vi "PES delay Mihai_March 2 2016 Brett1a.vi"(5 "Set velocity":string="200000") -> ()   [LabVIEW 2016]
uses:
  <vilib>/Waveform/WDTFileIO.llb/Export Waveforms To Spreadsheet File (1D).vi
  <vilib>/Instr/_visa.llb/VISA Configure Serial Port (Instr).vi
  <vilib>/Waveform/WDTFileIO.llb/Export Waveform To Spreadsheet File.vi
panel:
  out "Response 3":string="OK"
  out "Error 4":i32
  in  "Module # 3":i16
  out "Error 2":i32
  in  "Module # 4":i16
  out "Error 3":i32
  out "concatenated string 2":string="MA -21424\r"
  out "number 2":dbl=-21164.0
  out "return count 7":u32=15
  out "concatenated string":string="MA    104762\r"
  out "return count 5":u32=15
  out "read buffer 5":string="P:-0007564095\r\n"
  out "return count 4":u32
  out "return count 3":u32=15
  out "return count":u32
  out "read buffer":string
  in  "Resource Name":refnum<visa-resource-name>="COM1"
  in  "Baud Rate (9600)":u32=9600
  out "Error Information":errorcluster
  out "RoiSum":dbl=1786426.0
  out "ps 2":dbl=9.99159 format="%#_10g"
  out "coerced(x)":dbl=-2.22222
  out "P7887Sts Error":i32
  out "P7887Dat Error":i32
  out "TotalSum":dbl=1790796.0
  out "decimal integer string 2":string="MA -21424"
  out "Steps":dbl=-21423.532738095226 format="%.3f"
  out "mm 2":string="P:-0000021164\r\n"
  in  "offset 2":i32=2
  in  "Module # 2":i16
  out "Response 2":string="OK"
  in  "Tab Control 2":T1(tab)=enum."Measure PES"
  in  "offset":i32=2
  in  "stop":bool
  in  "Tab Control":enum32{"Setings", "Move / Measure"}(tab)=enum."Move / Measure"
  out "String":string="SV200000"
  out "number":dbl=104670.0
  out "go to new":string="    104762"
  out "ps":dbl=10.990350000000001 format="%#_10g"
  in  "ps":dbl=11.0
  out "Steps":dbl=104761.90476190475 format="%.3f"
  out "STEPS":string="P:+0000104670\r\n"
  in  "Radio Buttons":T2(radio)=enum."Radio Selection 4"
  in  "Boolean":bool=TRUE
  out "Status 3":T3={"Running"=1, "Runtime"=200.172, "TotalSum"=1790796.0, "RoiSum"=1786426.0, "RoiRate"=9885.0, "Fifo full"=0.0, "Sweeps"=199118.0, "Start events"=199118.0, "Maxval"=0} {"Fifo full" format="%.2f"; "Sweeps" format="%.2f"; "Start events" format="%.2f"; "RoiRate" format="%.2f"; "RoiSum" format="%.2f"; "TotalSum" format="%.2f"; "Runtime" format="%.2f"}
  in  "Transient Destination":path=path "C:/Documents and Settings/admin/My Documents/PES/2016/160310/T1_800+800nm.txt"
  out "XY Graph":T4(graph)=[{"Current position"=1.77597, "TotalSum"=1804610.0, "RoiSum"=1800421.0}, {"Current position"=1.5232350000000001, "TotalSum"=1788425.0, "RoiSum"=1783863.0}, {"Current position"=1.27617, "TotalSum"=1802098.0, "RoiSum"=1797659.0}, {"Current position"=1.023435, "TotalSum"=1791426.0, "RoiSum"=1786595.0}, {"Current position"=0.7745850000000001, "TotalSum"=1787483.0, "RoiSum"=1782845.0}, {"Current position"=0.52521, "TotalSum"=1821808.0, "RoiSum"=1817193.0}, {"Current position"=0.27604500000000004, "TotalSum"=1814052.0, "RoiSum"=1809669.0}, {"Current position"=0.027615, "TotalSum"=1806153.0, "RoiSum"=1801377.0}, {"Current position"=-0.22995000000000002, "TotalSum"=1812902.0, "RoiSum"=1808127.0}, {"Current position"=-0.47418000000000005, "TotalSum"=1823284.0, "RoiSum"=1818381.0}, {"Current position"=-0.728175, "TotalSum"=1800762.0, "RoiSum"=1796036.0}, {"Current position"=-0.9750300000000001, "TotalSum"=1812486.0, "RoiSum"=1807331.0}, {"Current position"=-1.222305, "TotalSum"=1825573.0, "RoiSum"=1821216.0}, {"Current position"=-1.46937, "TotalSum"=1829525.0, "RoiSum"=1824666.0}, {"Current position"=-1.721055, "TotalSum"=1840480.0, "RoiSum"=1835769.0}, {"Current position"=-1.96938, "TotalSum"=1820091.0, "RoiSum"=1815294.0}]
  out "x-y 2":dbl=-3.991535
  in  "No of steps":sgl=20.0 min=1 step=1
  in  "End":dbl=-10.0
  out "Begin":dbl=1.991535
  out "PS per step":dbl=-0.2494709375 min=1.0 max=10.0 step=1.0 format="%#_8g"
  out "Current position":dbl=-2.22222 format="%#_10g"
  out "appended path":path=path "C:/Documents and Settings/admin/My Documents/PES/2016/160310/2 TO -2 PS/2 TO -2/-2_22E+0.dat"
  in  "Photoelectron Spectra Destination":path=path "C:/Documents and Settings/admin/My Documents/PES/2016/160310/10 to -10/1_02E+0.dat"
  in  "No of Sweeps":dbl=199000.0
  out "Actual":dbl=199118.0
  in  "Module #":i16
  out "Settings P7887":T5={"Range"=6528, "Prena"=16, "Single sweeps"=39321856, "RoiMin"=2000, "RoiMax"=6500, "Roipreset"=0.0, "Timepreset"=1000.0, "SaveData"=0, "Format"=0, "Increm. Name"=FALSE, "Cycles"=2, "Sweep mode"=672, "Sync Out"=768, "Bitshift"=0, "Digval"=0, "Digio"=0, "DAC01"=29568, "DAC23"=31488, "SweepPreset"=200000.0, "#Regions"=0, "Caluse"=1, "First channel"=0.0, "Active"=1, "Calpoints"=0} {"DAC23" format="%.0x"; "DAC01" format="%.0x"; "Digio" format="%.0x"; "Sweep mode" format="%.0x"; "Prena" format="%.0x"; "First channel" format="%.2f"; "Sync Out" format="%.0x"; "SweepPreset" format="%.2f"; "SaveData" format="%.0x"; "Timepreset" format="%.2f"; "Roipreset" format="%.2f"}
  out "Data":u32[](graph)
  out "position set":dbl=-2.249470937499999 min=1.0 max=10.0 step=1.0 format="%#_8g"
  in  "Status":T6(radio)=enum."Finish recorging S#"
  # "Delay"
  # "Delay"
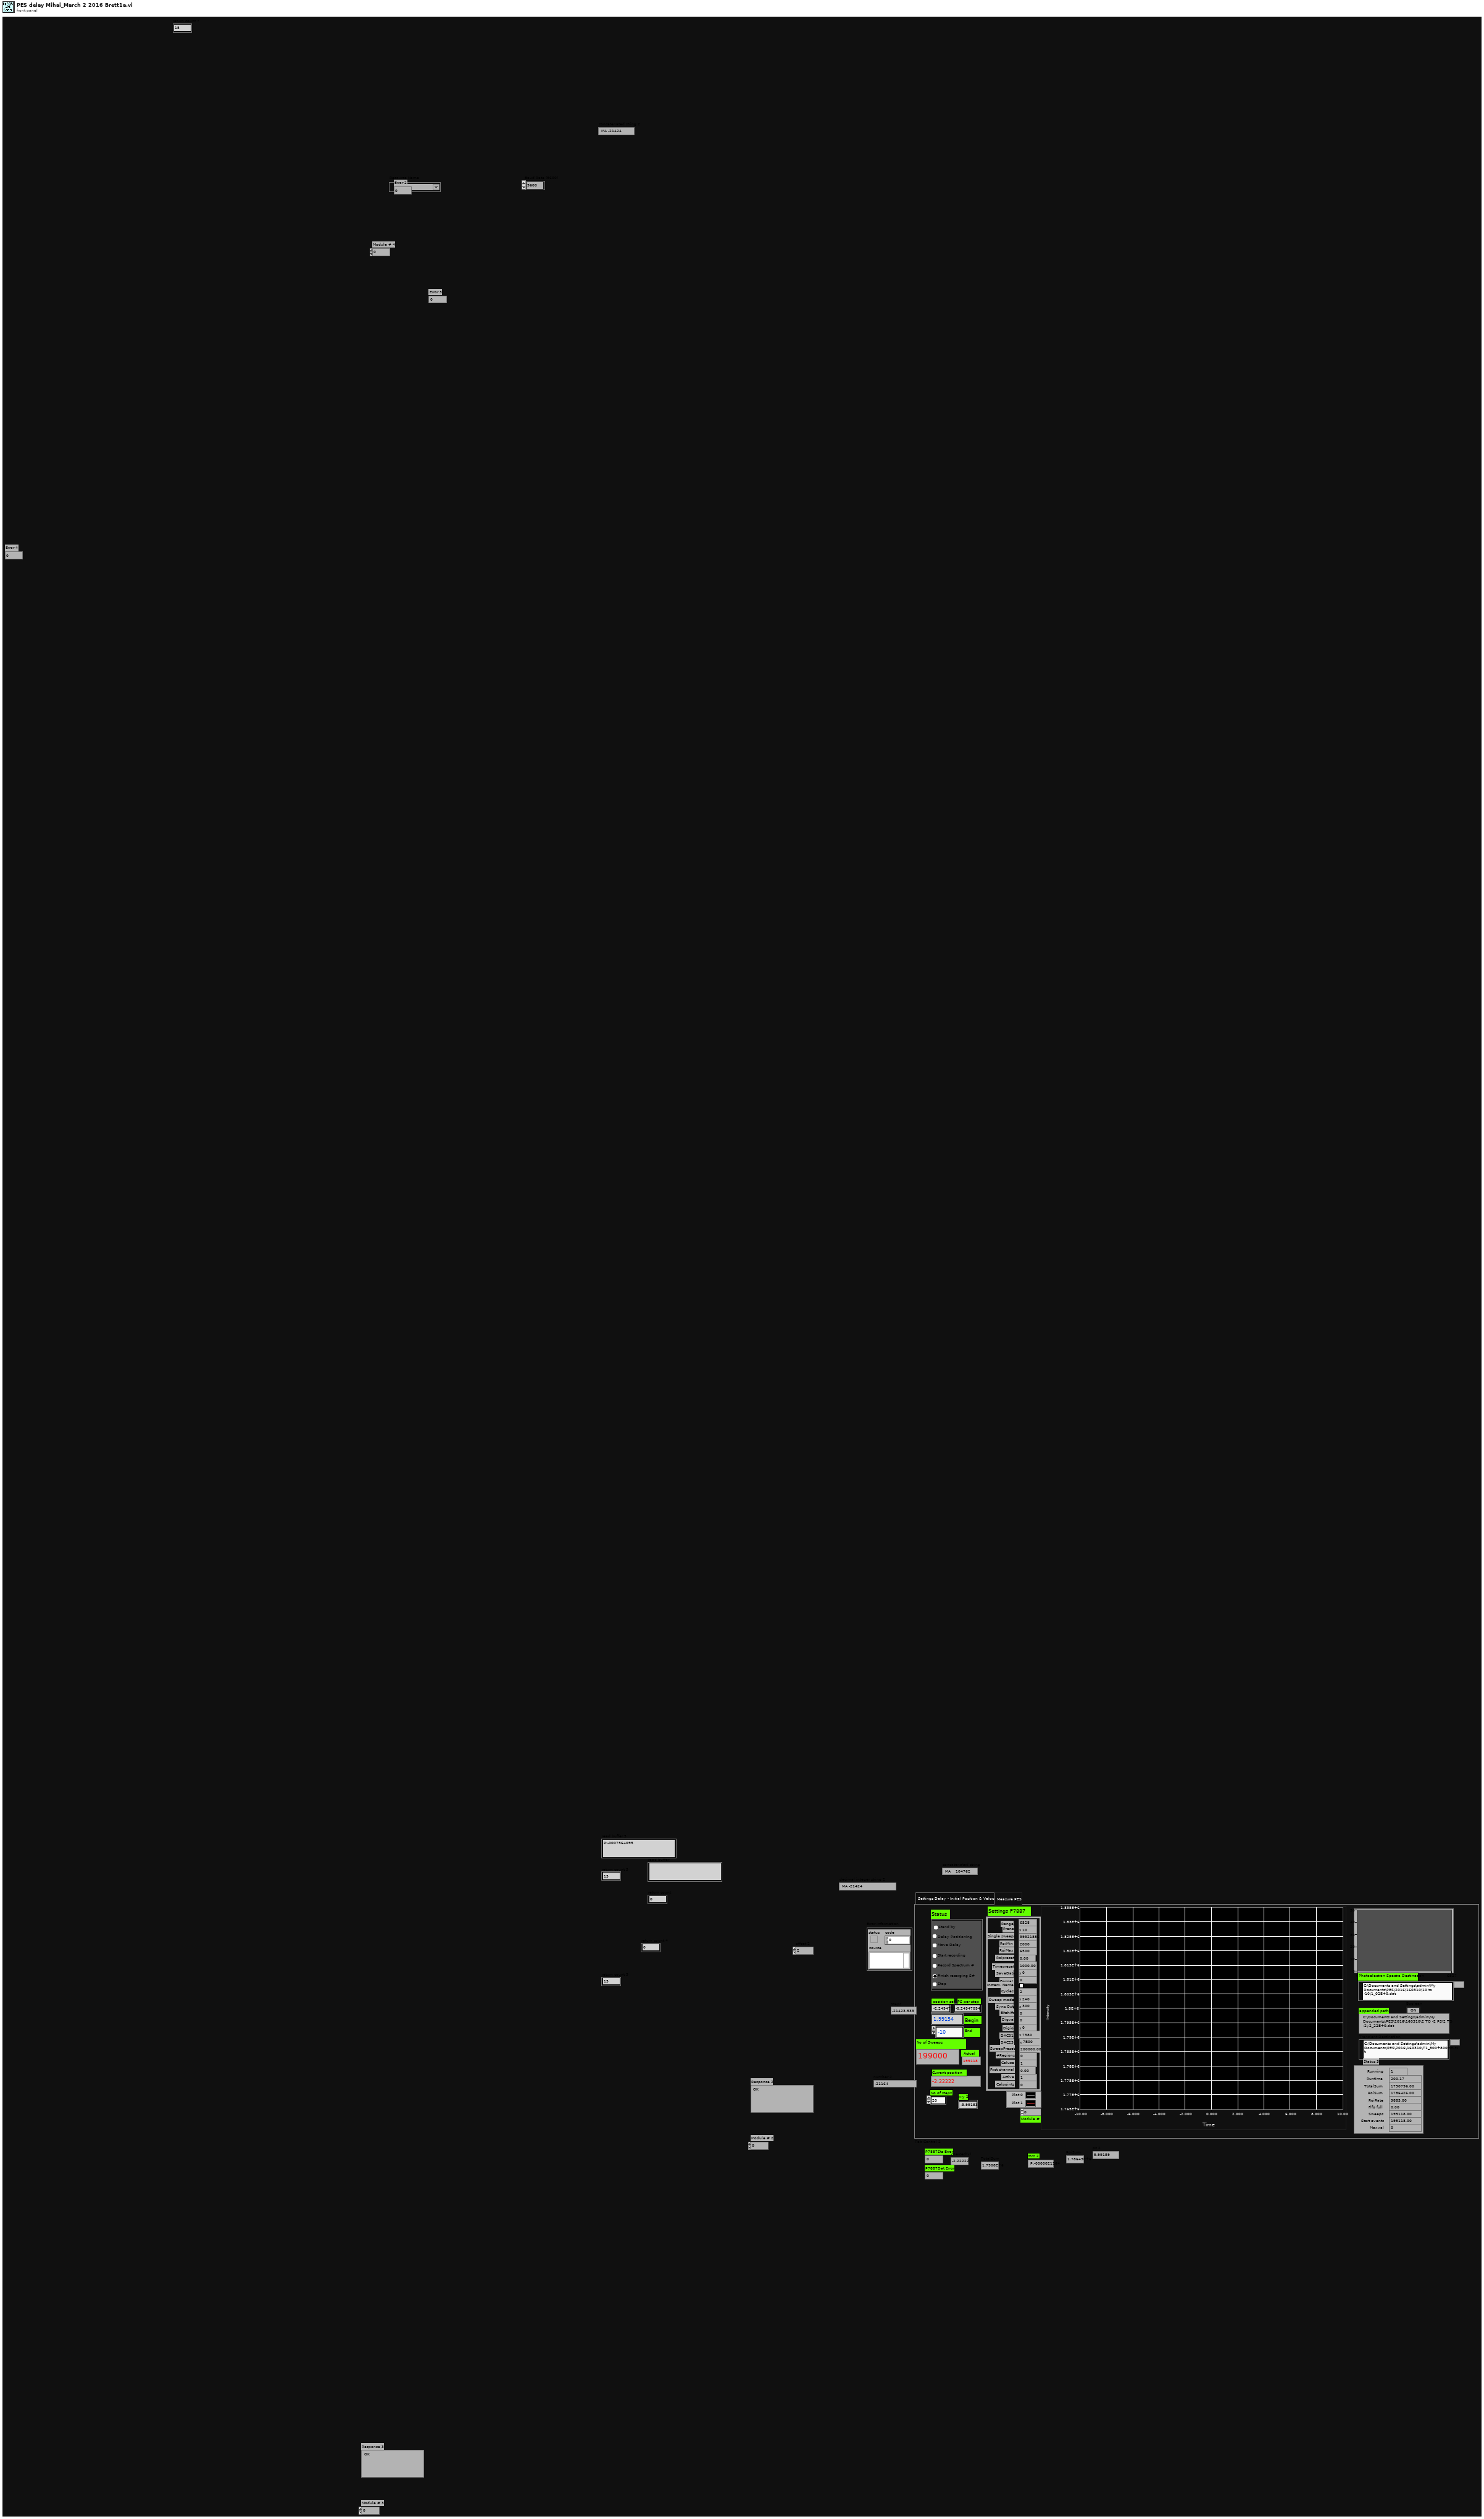
[diagram p1: front panel]
types:
  T1 = enum32{"Settings Delay - Initial Pozition & Velocity", "Measure PES"}
  T2 = enum32{"Stop", "Radio Selection 2", "Radio Selection 3", "Radio Selection 4"}
  T3 = cluster{"Running":i32, "Runtime":dbl, "TotalSum":dbl, "RoiSum":dbl, "RoiRate":dbl, "Fifo full":dbl, "Sweeps":dbl, "Start events":dbl, "Maxval":u32}
  T4 = cluster{"Current position":dbl, "TotalSum":dbl, "RoiSum":dbl}[]
  T5 = cluster{"Range":i32, "Prena":u32, "Single sweeps":u32, "RoiMin":u32, "RoiMax":u32, "Roipreset":dbl, "Timepreset":dbl, "SaveData":u32, "Format":i32, "Increm. Name":bool, "Cycles":u32, "Sweep mode":u32, "Sync Out":u32, "Bitshift":i32, "Digval":u32, "Digio":u32, "DAC01":u32, "DAC23":u32, "SweepPreset":dbl, "#Regions":i32, "Caluse":i32, "First channel":dbl, "Active":i32, "Calpoints":i32}
  T6 = enum32{"Delay Pozitioning", "Move Delay", "Record Spectrum #", "Finish recorging S#", "Stop ", "Start recording", "Stand by"}
  T7 = enum32{"Delay Pozitioning", "Move Delay", "Record Spectrum #", "Finish recorging S#", "Stop", "Start recording", "Stand by"}
  T8 = cluster{"Range":i32, "Prena":u32, "Cftfak":i32, "RoiMin":u32, "RoiMax":u32, "Roipreset":dbl, "Timepreset":dbl, "SaveData":u32, "Format":i32, "Increm. Name":bool, "Cycles":u32, "Sweep mode":u32, "Sync Out":u32, "Bitshift":i32, "Digval":u32, "Digio":u32, "DAC0":u32, "DAC1":u32, "SweepPreset":dbl, "#Regions":i32, "Caluse":i32, "First channel":dbl, "Active":i32, "Calpoints":i32}
  T9 = cluster{"Current position":dbl, "TotalSum":dbl, "RoiSum":dbl}
  T10 = cluster{waveform(dbl), waveform(dbl), waveform(dbl)}
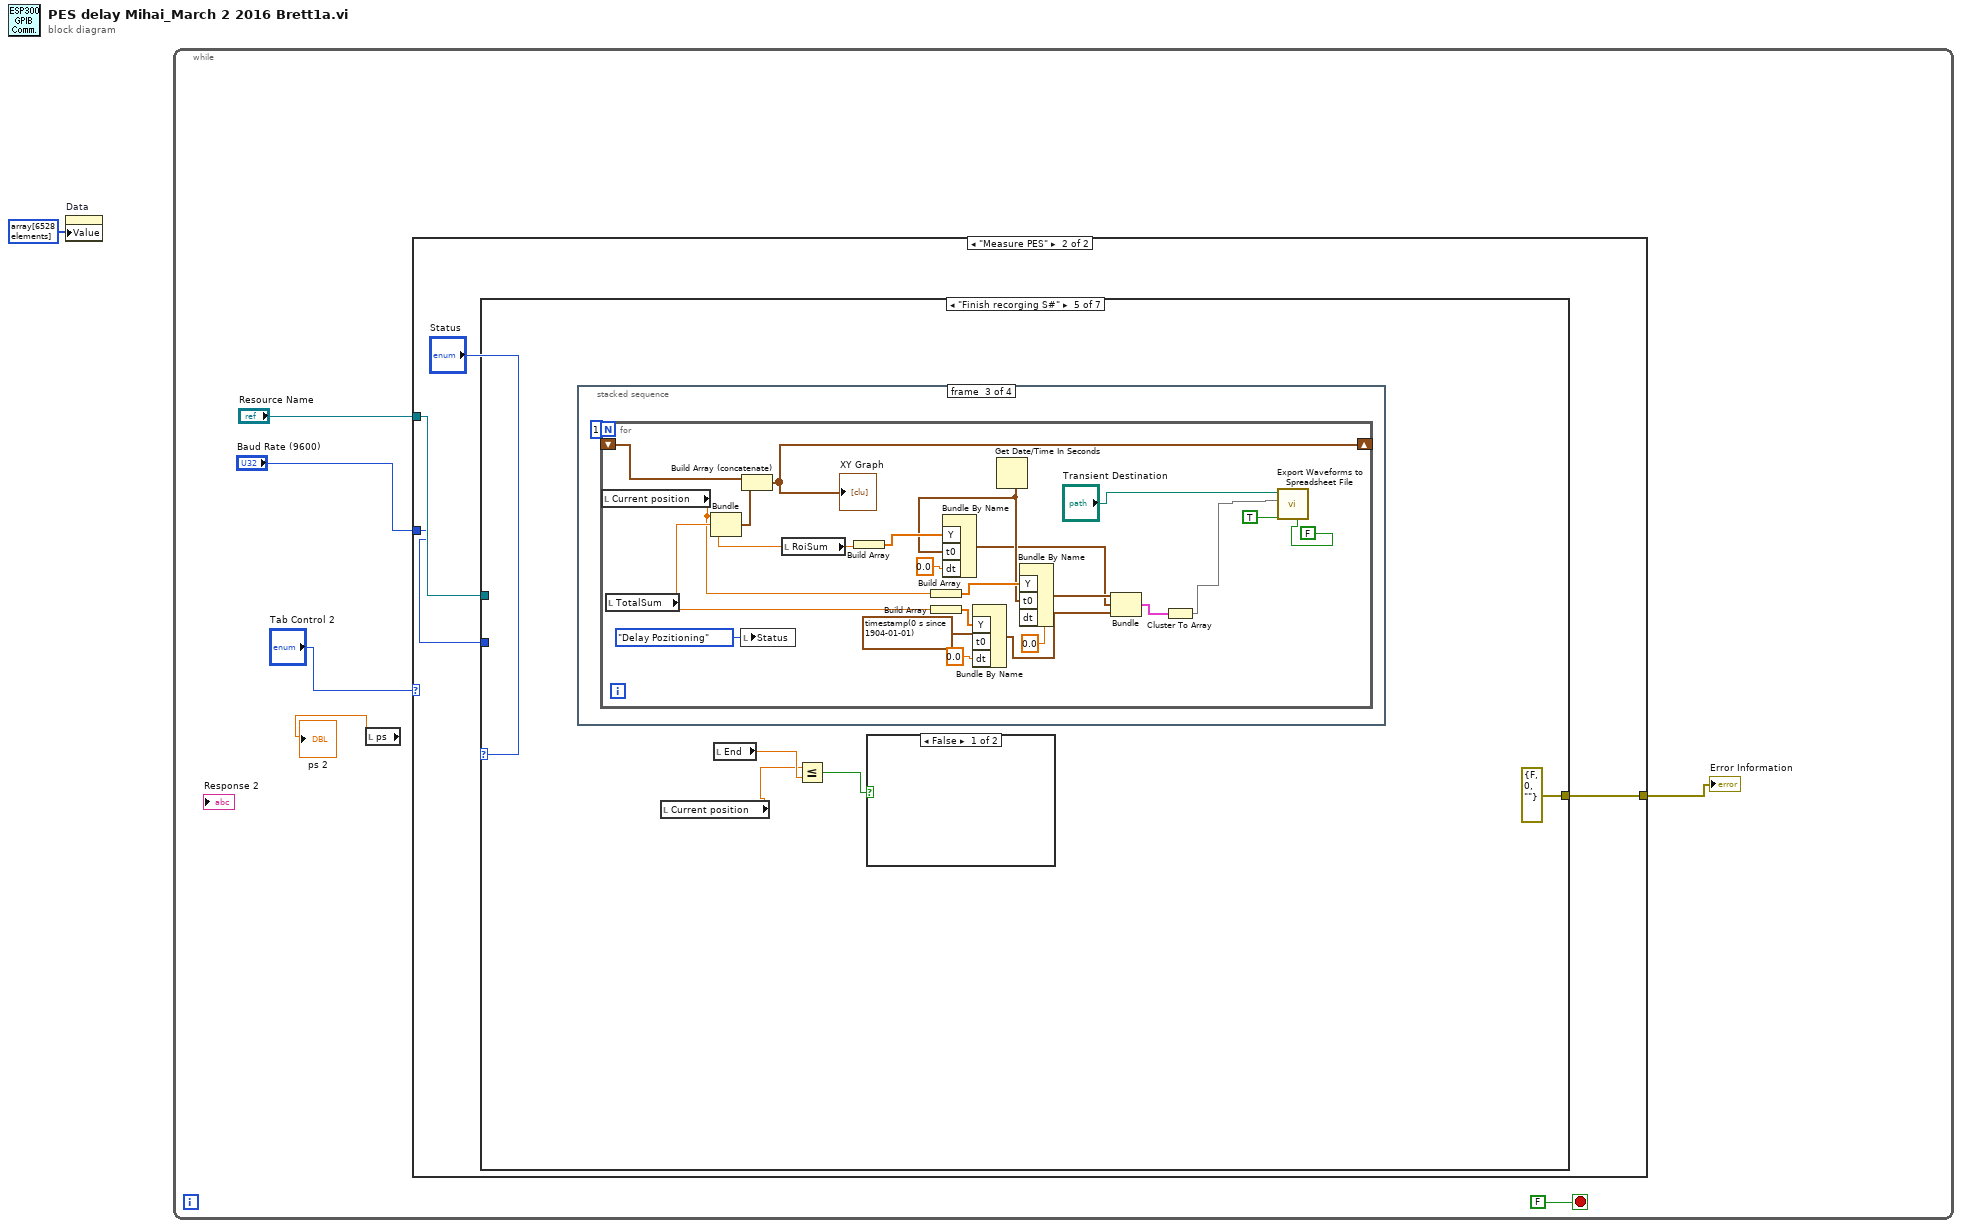
[diagram p0: block diagram]
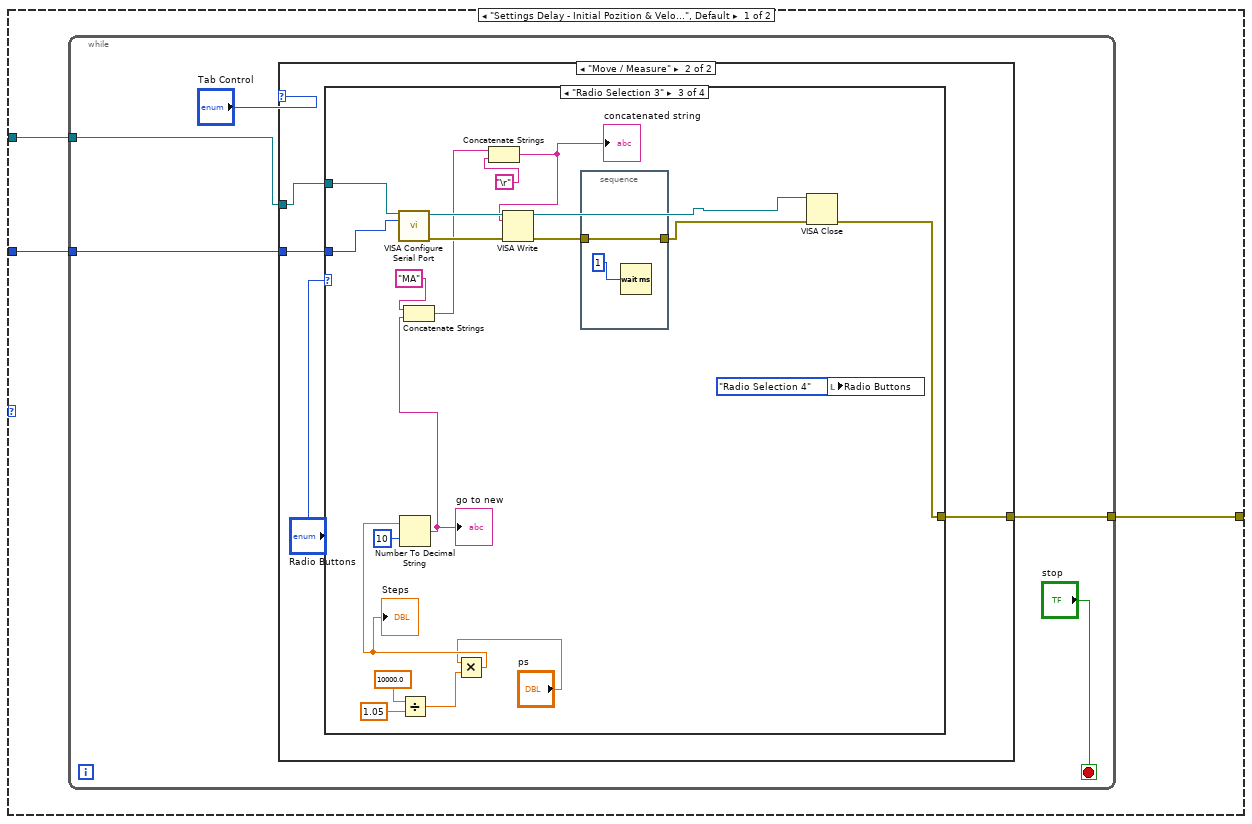
[diagram p2: hidden frame]
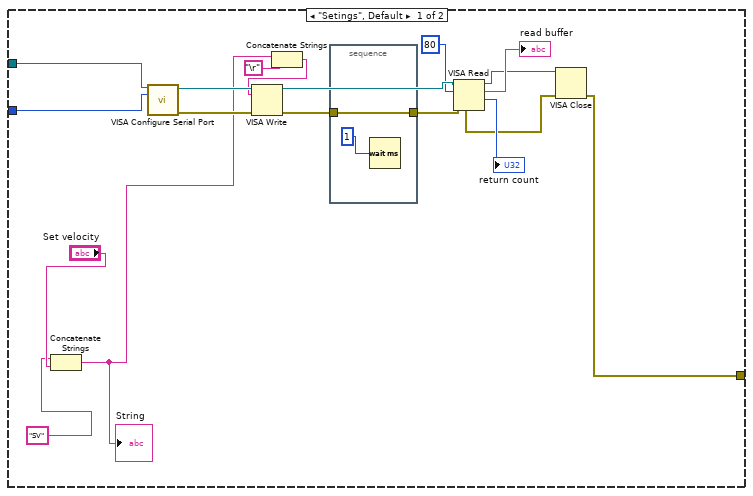
[diagram p3: hidden frame]
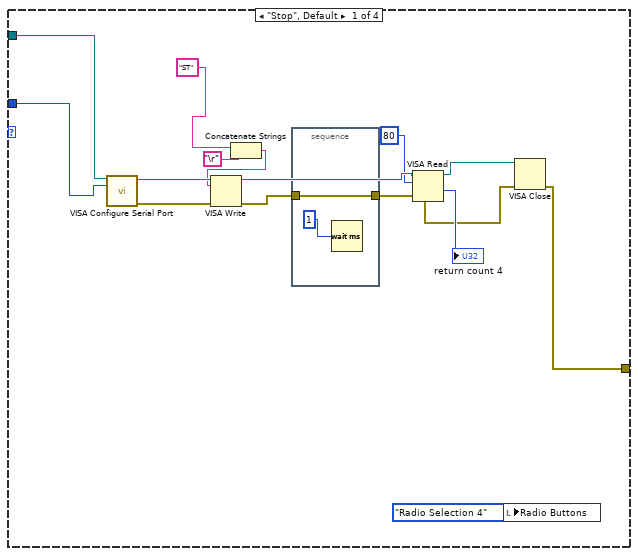
[diagram p4: hidden frame]
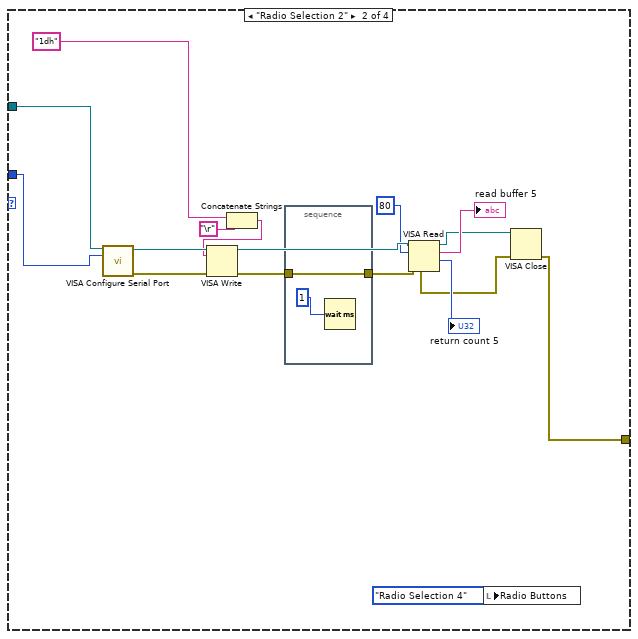
[diagram p5: hidden frame]
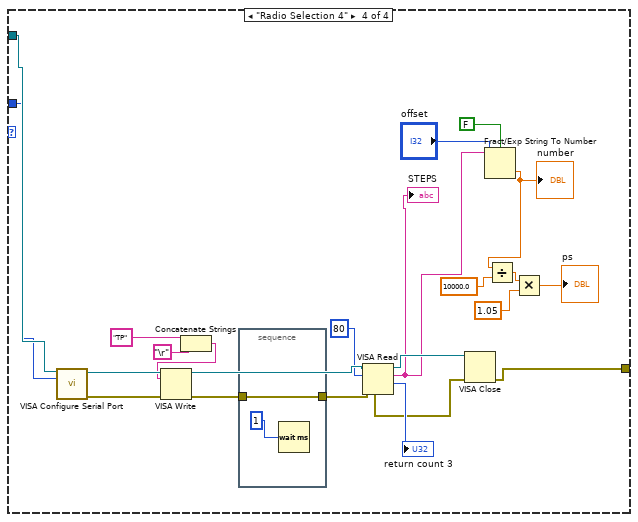
[diagram p6: hidden frame]
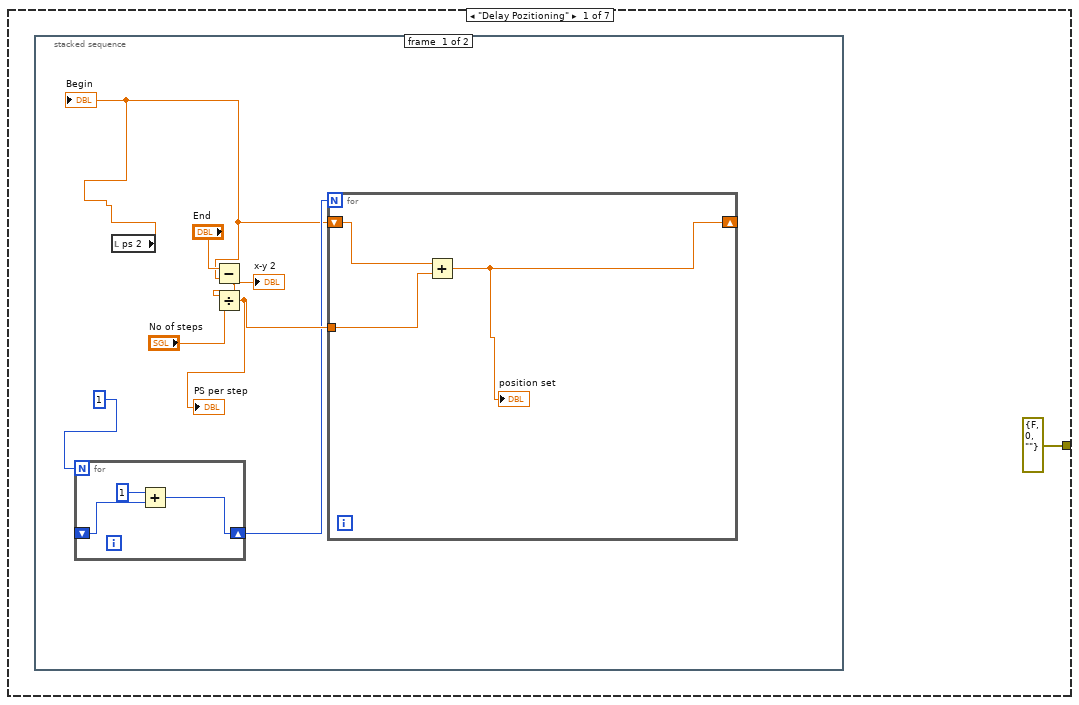
[diagram p7: hidden frame]
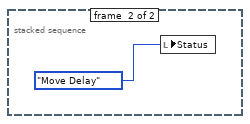
[diagram p8: hidden frame]
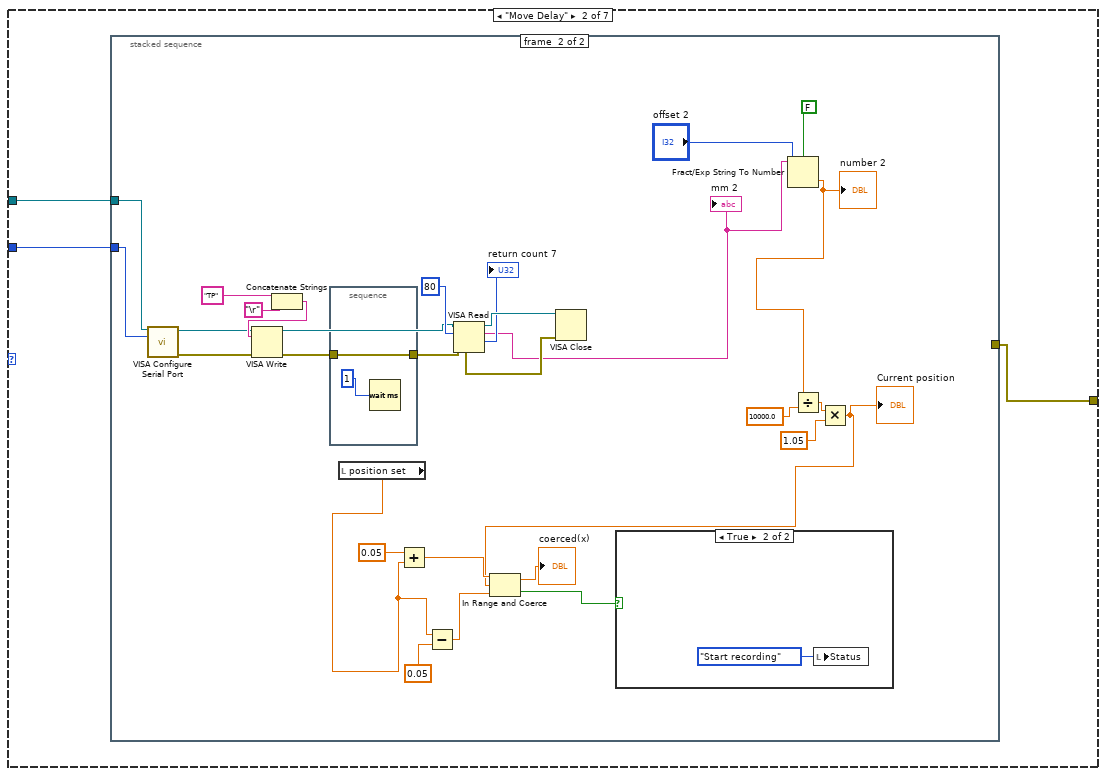
[diagram p9: hidden frame]
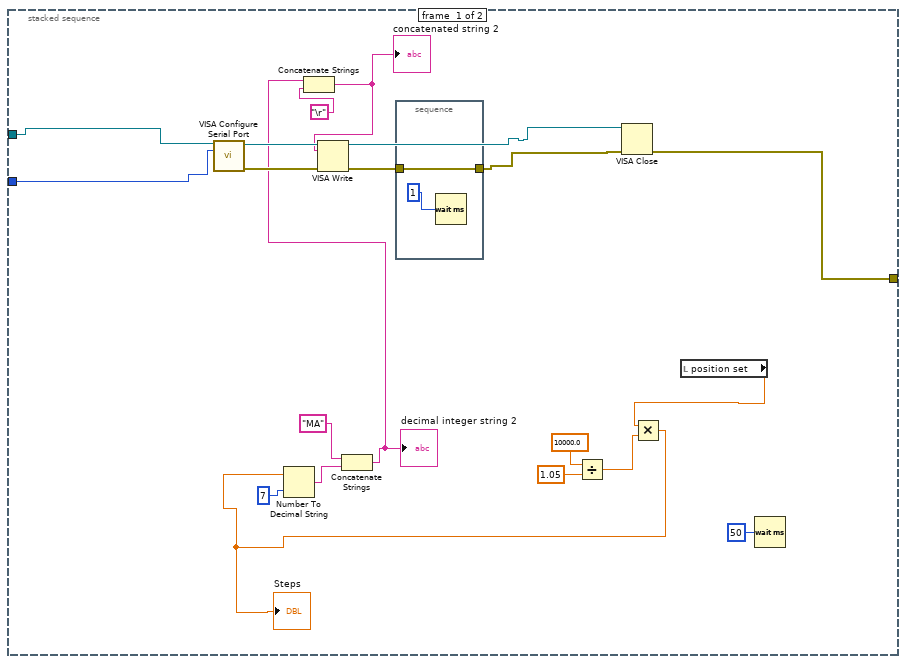
[diagram p10: hidden frame]
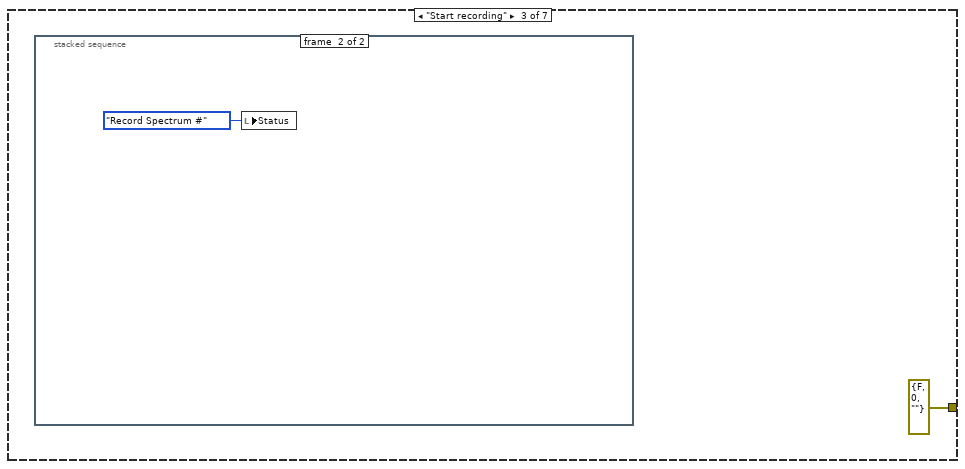
[diagram p12: hidden frame]
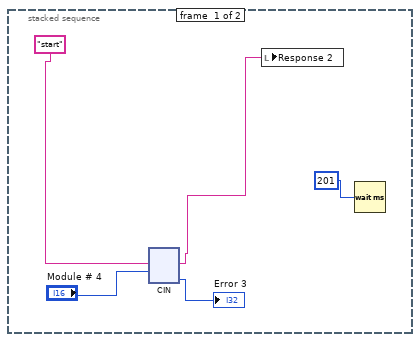
[diagram p13: hidden frame]
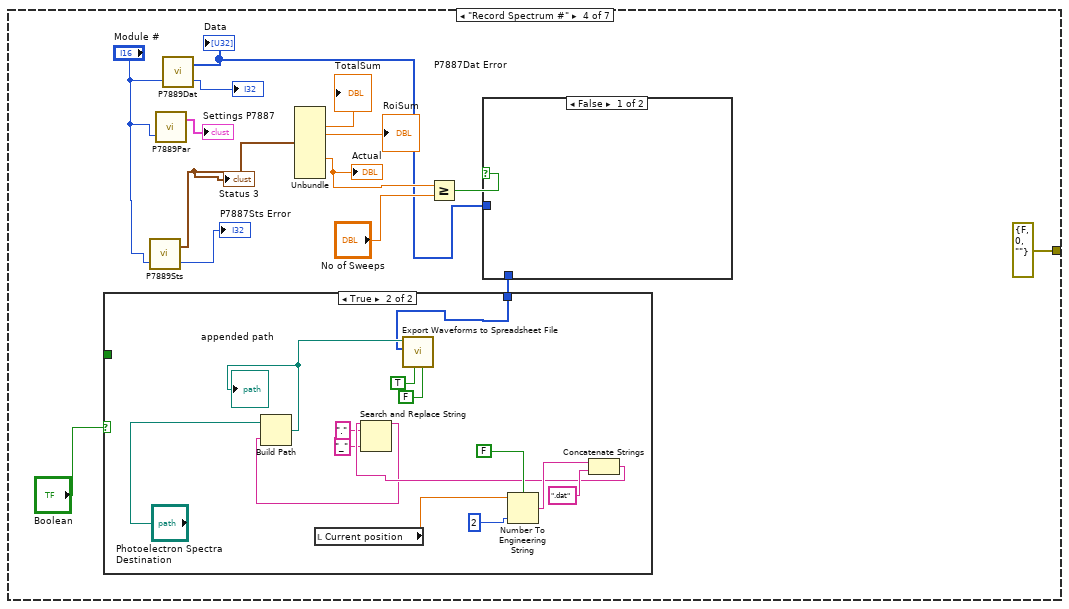
[diagram p14: hidden frame]
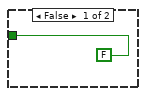
[diagram p15: hidden frame]
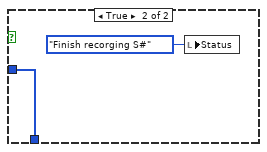
[diagram p16: hidden frame]
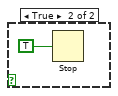
[diagram p17: hidden frame]
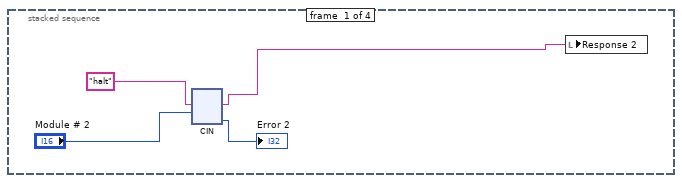
[diagram p18: hidden frame]
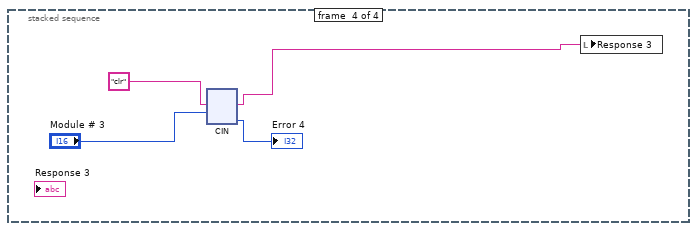
[diagram p20: hidden frame]
diagram:
  n1 = property on="Data" class="WFGraph (strict)"("Value"=u32[] array[6528 elements] ("Data")) -> ()  [unwired: 2 in, 2 out]
  n2 = while {
    stop <- FALSE stop-if-true
    n3 = local read "ps"() -> (→"ps 2":dbl)
    n4 = case shown="\"Measure PES\"" "Tab Control 2" {
      tunnel: "Resource Name" -> [w10 w125]
      tunnel: "Baud Rate (9600)" -> [w9 w124]
      tunnel: [w8 w126] -> w2
      frame "Settings Delay - Initial Pozition & Velocity", Default {
        n5 = while {
          tunnel: w10 -> [w13]
          tunnel: w9 -> [w12]
          tunnel: [w11] -> w8
          stop <- "stop" stop-if-true
          n6 = case shown="\"Move / Measure\"" "Tab Control" {
            tunnel: [w19 w36] -> w11
            tunnel: w13 -> [w18 w38]
            tunnel: w12 -> [w17 w37]
            frame "Setings", Default {
              n7 = Concatenate Strings("SV" ("string"), "Set velocity") -> (w16:string)
              "String" <- w16
              n8 = call-poly "VISA Configure Serial Port"("VISA resource name"=w18, "baud rate (9600)"=w17) -> ("VISA resource name out"=w30:refnum<visa-resource-name>, "error out"=w31:errorcluster)  [unwired: 12 in]
              n9 = Concatenate Strings(w16, "\r") -> (w22:string)
              n10 = VISA Write(VISA resource name=w30, write buffer=w22, error in (no error)=w31) -> (VISA resource name out=w29:refnum<visa-resource-name>, error out=w27:errorcluster)  [unwired: 1 out]
              n11 = stacked-sequence {
                tunnel: w27 -> [w34]
                tunnel: [w34] -> w26
                frame #0 {
                  n12 = Wait (ms)(milliseconds to wait=u32 1) -> ()  [unwired: 1 out]
                }
              }
              n13 = VISA Read(VISA resource name=w29, byte count=u32 80 ("byte count (0)"), error in (no error)=w26) -> (VISA resource name out=w21:refnum<visa-resource-name>, read buffer=→"read buffer":string, return count=→"return count":u32, error out=w20:errorcluster)
              n14 = VISA Close(VISA resource name=w21, error in (no error)=w20) -> (error out=w19:errorcluster)
            }
            frame "Move / Measure" {
              n15 = case shown="\"Radio Selection 3\"" "Radio Buttons" {
                tunnel: w38 -> [w42 w60 w83 w107]
                tunnel: w37 -> [w41 w58 w82 w106]
                tunnel: [w40 w61 w80 w104] -> w36
                frame "Stop", Default {
                  n16 = call-poly "VISA Configure Serial Port"("VISA resource name"=w42, "baud rate (9600)"=w41) -> ("VISA resource name out"=w53:refnum<visa-resource-name>, "error out"=w54:errorcluster)  [unwired: 12 in]
                  n17 = Concatenate Strings("ST" ("Set velocity 2"), "\r") -> (w46:string)
                  n18 = VISA Write(VISA resource name=w53, write buffer=w46, error in (no error)=w54) -> (VISA resource name out=w52:refnum<visa-resource-name>, error out=w50:errorcluster)  [unwired: 1 out]
                  n19 = stacked-sequence {
                    tunnel: w50 -> [w56]
                    tunnel: [w56] -> w49
                    frame #0 {
                      n20 = Wait (ms)(milliseconds to wait=u32 1) -> ()  [unwired: 1 out]
                    }
                  }
                  n21 = VISA Read(VISA resource name=w52, byte count=u32 80 ("byte count (0)"), error in (no error)=w49) -> (VISA resource name out=w45:refnum<visa-resource-name>, return count=→"return count 4":u32, error out=w44:errorcluster)  [unwired: 1 out]
                  n22 = local write "Radio Buttons"(T2."Radio Selection 4" ("Radio Buttons")) -> ()
                  n23 = VISA Close(VISA resource name=w45, error in (no error)=w44) -> (error out=w40:errorcluster)
                }
                frame "Radio Selection 2" {
                  n24 = call-poly "VISA Configure Serial Port"("VISA resource name"=w60, "baud rate (9600)"=w58) -> ("VISA resource name out"=w72:refnum<visa-resource-name>, "error out"=w73:errorcluster)  [unwired: 12 in]
                  n25 = Concatenate Strings("1dh" ("Set velocity 2"), "\r") -> (w64:string)
                  n26 = VISA Write(VISA resource name=w72, write buffer=w64, error in (no error)=w73) -> (VISA resource name out=w71:refnum<visa-resource-name>, error out=w69:errorcluster)  [unwired: 1 out]
                  n27 = stacked-sequence {
                    tunnel: w69 -> [w75]
                    tunnel: [w75] -> w68
                    frame #0 {
                      n28 = Wait (ms)(milliseconds to wait=u32 1) -> ()  [unwired: 1 out]
                    }
                  }
                  n29 = VISA Read(VISA resource name=w71, byte count=u32 80 ("byte count (0)"), error in (no error)=w68) -> (VISA resource name out=w63:refnum<visa-resource-name>, read buffer=→"read buffer 5":string, return count=→"return count 5":u32, error out=w62:errorcluster)
                  n30 = local write "Radio Buttons"(T2."Radio Selection 4" ("Radio Buttons")) -> ()
                  n31 = VISA Close(VISA resource name=w63, error in (no error)=w62) -> (error out=w61:errorcluster)
                }
                frame "Radio Selection 3" {
                  n32 = call-poly "VISA Configure Serial Port"("VISA resource name"=w83, "baud rate (9600)"=w82) -> ("VISA resource name out"=w87:refnum<visa-resource-name>, "error out"=w88:errorcluster)  [unwired: 12 in]
                  n33 = Divide(x=10000.0 ("y"), y=1.05) -> (x/y=w90:dbl)
                  n34 = Multiply(x="ps", y=w90) -> (x*y=w93:dbl)
                  "Steps" <- w93
                  n35 = Number To Decimal String(number=w93, width (-)=i16 10) -> (decimal integer string=w79:string)
                  "go to new" <- w79
                  n36 = Concatenate Strings("MA" ("Set velocity 2"), w79) -> (w81:string)
                  n37 = Concatenate Strings(w81, "\r") -> (w84:string)
                  "concatenated string" <- w84
                  n38 = VISA Write(VISA resource name=w87, write buffer=w84, error in (no error)=w88) -> (VISA resource name out=w78:refnum<visa-resource-name>, error out=w86:errorcluster)  [unwired: 1 out]
                  n39 = stacked-sequence {
                    tunnel: w86 -> [w97]
                    tunnel: [w97] -> w77
                    frame #0 {
                      n40 = Wait (ms)(milliseconds to wait=u32 1) -> ()  [unwired: 1 out]
                    }
                  }
                  n41 = VISA Close(VISA resource name=w78, error in (no error)=w77) -> (error out=w80:errorcluster)
                  n42 = local write "Radio Buttons"(T2."Radio Selection 4" ("Radio Buttons")) -> ()
                }
                frame "Radio Selection 4" {
                  n43 = call-poly "VISA Configure Serial Port"("VISA resource name"=w107, "baud rate (9600)"=w106) -> ("VISA resource name out"=w117:refnum<visa-resource-name>, "error out"=w118:errorcluster)  [unwired: 12 in]
                  n44 = Concatenate Strings("TP" ("Set velocity 2"), "\r") -> (w110:string)
                  n45 = VISA Write(VISA resource name=w117, write buffer=w110, error in (no error)=w118) -> (VISA resource name out=w116:refnum<visa-resource-name>, error out=w114:errorcluster)  [unwired: 1 out]
                  n46 = stacked-sequence {
                    tunnel: w114 -> [w122]
                    tunnel: [w122] -> w113
                    frame #0 {
                      n47 = Wait (ms)(milliseconds to wait=u32 1) -> ()  [unwired: 1 out]
                    }
                  }
                  n48 = VISA Read(VISA resource name=w116, byte count=u32 80 ("byte count (0)"), error in (no error)=w113) -> (VISA resource name out=w109:refnum<visa-resource-name>, read buffer=w103:string, return count=→"return count 3":u32, error out=w108:errorcluster)
                  "STEPS" <- w103
                  n49 = VISA Close(VISA resource name=w109, error in (no error)=w108) -> (error out=w104:errorcluster)
                  n50 = Fract/Exp String To Number(use system decimal point (T)=FALSE, string=w103, offset="offset") -> (number=w119:dbl)  [unwired: 1 in, 1 out]
                  "number" <- w119
                  n51 = Divide(x=w119, y=10000.0) -> (x/y=w101:dbl)
                  n52 = Multiply(x=w101, y=1.05) -> (x*y=→"ps":dbl)
                }
              }
            }
          }
        }
      }
      frame "Measure PES" {
        n53 = case shown="\"Finish recorging S#\"" "Status" {
          tunnel: [errorcluster {"status"=FALSE, "code"=0, "source"=""} ("error out") w145 errorcluster {"status"=FALSE, "code"=0, "source"=""} ("error out") errorcluster {"status"=FALSE, "code"=0, "source"=""} ("error out") errorcluster {"status"=FALSE, "code"=0, "source"=""} ("error out") errorcluster {"status"=FALSE, "code"=0, "source"=""} ("error out") errorcluster {"status"=FALSE, "code"=0, "source"=""} ("error out")] -> w126
          tunnel: w125 -> [_ w144 _ _ _ _ _]
          tunnel: w124 -> [_ w143 _ _ _ _ _]
          frame "Delay Pozitioning" {
            n54 = stacked-sequence {
              frame #0 {
                n55 = for {
                  N: 1 -> [_]
                  shift-right: [w136] -> w132
                  shift-left: _ -> [w138]
                  n56 = Add(x=1, y=w138) -> (x+y=w136:i32)
                }
                n57 = local read "ps 2"() -> (w129:dbl)
                "Begin" <- w129
                n58 = Subtract(x="End", y=w129) -> (x-y=w135:dbl)
                "x-y 2" <- w135
                n59 = Divide(x=w135, y="No of steps") -> (x/y=w134:dbl)
                "PS per step" <- w134
                n60 = for {
                  N: w132 -> [_]
                  shift-right: [w139] -> _
                  shift-left: w129 -> [w141]
                  tunnel: w134 -> [w140]
                  n61 = Add(x=w141, y=w140) -> (x+y=w139:dbl)
                  "position set" <- w139
                }
              }
              frame #1 {
                n62 = local write "Status"(T7."Move Delay" ("Status")) -> ()
              }
            }
          }
          frame "Move Delay" {
            n63 = stacked-sequence {
              tunnel: w144 -> [w151 w170]
              tunnel: w143 -> [w150 w169]
              tunnel: [w149 _] -> w145
              frame #0 {
                n64 = call-poly "VISA Configure Serial Port"("VISA resource name"=w151, "baud rate (9600)"=w150) -> ("VISA resource name out"=w155:refnum<visa-resource-name>, "error out"=w156:errorcluster)  [unwired: 12 in]
                n65 = Divide(x=10000.0 ("y"), y=1.05) -> (x/y=w162:dbl)
                n66 = local read "position set"() -> (w161:dbl)
                n67 = Multiply(x=w161, y=w162) -> (x*y=w157:dbl)
                "Steps" <- w157
                n68 = Number To Decimal String(number=w157, width (-)=i16 7) -> (decimal integer string=w159:string)
                n69 = Concatenate Strings("MA" ("Set velocity 2"), w159) -> (w148:string)
                "decimal integer string 2" <- w148
                n70 = Concatenate Strings(w148, "\r") -> (w152:string)
                "concatenated string 2" <- w152
                n71 = VISA Write(VISA resource name=w155, write buffer=w152, error in (no error)=w156) -> (VISA resource name out=w147:refnum<visa-resource-name>, error out=w154:errorcluster)  [unwired: 1 out]
                n72 = stacked-sequence {
                  tunnel: w154 -> [w166]
                  tunnel: [w166] -> w146
                  frame #0 {
                    n73 = Wait (ms)(milliseconds to wait=u32 1) -> ()  [unwired: 1 out]
                  }
                }
                n74 = VISA Close(VISA resource name=w147, error in (no error)=w146) -> (error out=w149:errorcluster)
                n75 = Wait (ms)(milliseconds to wait=u32 50) -> ()  [unwired: 1 out]
              }
              frame #1 {
                n76 = call-poly "VISA Configure Serial Port"("VISA resource name"=w170, "baud rate (9600)"=w169) -> ("VISA resource name out"=w172:refnum<visa-resource-name>, "error out"=w171:errorcluster)  [unwired: 12 in]
                n77 = Concatenate Strings("TP" ("Set velocity 2"), "\r") -> (w179:string)
                n78 = VISA Write(VISA resource name=w172, write buffer=w179, error in (no error)=w171) -> (VISA resource name out=w173:refnum<visa-resource-name>, error out=w175:errorcluster)  [unwired: 1 out]
                n79 = stacked-sequence {
                  tunnel: w175 -> [w197]
                  tunnel: [w197] -> w176
                  frame #0 {
                    n80 = Wait (ms)(milliseconds to wait=u32 1) -> ()  [unwired: 1 out]
                  }
                }
                n81 = local read "position set"() -> (w188:dbl)
                n82 = Add(x=0.05, y=w188) -> (x+y=w192:dbl)
                n83 = Subtract(x=w188, y=0.05 ("x")) -> (x-y=w190:dbl)
                n84 = VISA Read(VISA resource name=w173, byte count=u32 80 ("byte count (0)"), error in (no error)=w176) -> (VISA resource name out=w180:refnum<visa-resource-name>, read buffer=w168:string, return count=→"return count 7":u32, error out=w181:errorcluster)
                "mm 2" <- w168
                n85 = VISA Close(VISA resource name=w180, error in (no error)=w181) -> ()  [unwired: 1 out]
                n86 = Fract/Exp String To Number(use system decimal point (T)=FALSE, string=w168, offset="offset 2") -> (number=w184:dbl)  [unwired: 1 in, 1 out]
                "number 2" <- w184
                n87 = Divide(x=w184, y=10000.0) -> (x/y=w186:dbl)
                n88 = Multiply(x=w186, y=1.05) -> (x*y=w183:dbl)
                "Current position" <- w183
                n89 = In Range and Coerce(upper limit=w192, x=w183, lower limit=w190) -> (coerced(x)=→"coerced(x)":dbl, In Range?=w194:bool)
                n90 = case shown="True" w194 {
                  frame False {
                  }
                  frame True {
                    n91 = local write "Status"(T7."Start recording" ("Status")) -> ()
                  }
                }
              }
            }
          }
          frame "Start recording" {
            n92 = stacked-sequence {
              frame #0 {
                n93 = cin("start" ("Command"), "Module # 4") -> (w202:string, →"Error 3":i32)  [unwired: 2 in]
                n94 = local write "Response 2"(w202) -> ()
                n95 = Wait (ms)(milliseconds to wait=u32 201) -> ()  [unwired: 1 out]
              }
              frame #1 {
                n96 = local write "Status"(T7."Record Spectrum #" ("Status")) -> ()
              }
            }
          }
          frame "Record Spectrum #" {
            n97 = call "P7889Sts.vi"("Module #"="Module #") -> ("P7889Sts Error"=→"P7887Sts Error":i32, "Status"=w213:T3)  [unwired: 1 in]
            "Status 3" <- w213
            n98 = call "P7889Par.vi"("Module #"="Module #") -> ("Settings"=→"Settings P7887":T8)  [unwired: 1 in, 1 out]
            n99 = call "P7889Dat.vi"("Module #"="Module #") -> ("P7889Dat Error"=→"P7887Dat Error":i32, "Data"=w208:u32[])  [unwired: 1 in]
            "Data" <- w208
            n100 = Unbundle(w213) -> ("TotalSum"=→"TotalSum":dbl, "RoiSum"=→"RoiSum":dbl, "Sweeps"=w210:dbl)  [unwired: 6 out]
            "Actual" <- w210
            n101 = Greater Or Equal?(x=w210, y="No of Sweeps") -> (x >= y?=w218:bool)
            n102 = case shown="False" w218 {
              tunnel: w208 -> [_ w236]
              tunnel: [_ w236] -> w207
              frame False {
              }
              frame True {
                n103 = local write "Status"(T7."Finish recorging S#" ("Status")) -> ()
              }
            }
            n104 = case shown="True" "Boolean" {
              tunnel: [FALSE ("Boolean 2") _] -> _
              tunnel: w207 -> [_ w222]
              frame False {
              }
              frame True {
                n105 = local read "Current position"() -> (w227:dbl)
                n106 = Number To Engineering String(1:FALSE ("use system decimal point (T)"), 2:i16 2 ("width (-)"), 4:w227) -> (0:w229:string)  [unwired: 1 in]
                n107 = Concatenate Strings(w229, ".dat" ("string")) -> (w226:string)
                n108 = Search and Replace String(input string=w226, search string=".", replace string="_" ("replace string (\"\")")) -> (result string=w223:string)  [unwired: 5 in, 3 out]
                n109 = Build Path(base path="Photoelectron Spectra Destination", name or relative path=w223) -> (appended path=w233:path)
                "appended path" <- w233
                n110 = call-poly <vilib>:"Export Waveforms to Spreadsheet File.vi"("header? (write header:T)"=FALSE ("Header? (write header:T)"), "append to file? (new file:F)"=TRUE, "waveform"=w222, "file path (dialog if empty)"=w233) -> ()  [unwired: 6 in, 2 out]
              }
            }
          }
          frame "Finish recorging S#" {
            n111 = stacked-sequence {
              frame #0 {
                n112 = cin("halt" ("Command"), "Module # 2") -> (w243:string, →"Error 2":i32)  [unwired: 2 in]
                n113 = local write "Response 2"(w243) -> ()
              }
              frame #1 {
              }
              frame #2 {
                n114 = for {
                  N: 1 -> [_]
                  shift-right: [w267] -> _
                  shift-left: _ -> [w268]
                  n115 = local read "Current position"() -> (w257:dbl)
                  n116 = local read "TotalSum"() -> (w258:dbl)
                  n117 = local write "Status"(T7."Delay Pozitioning" ("Status")) -> ()
                  n118 = local read "RoiSum"() -> (w252:dbl)
                  n119 = Bundle("Current position"=w257, "TotalSum"=w258, "RoiSum"=w252) -> (w269:T9)  [unwired: 1 in]
                  n120 = Build Array (concatenate)(w268, w269) -> (w267:T4)
                  "XY Graph" <- w267
                  n121 = Build Array(w252) -> (w253:dbl[])
                  n122 = Build Array(w257) -> (w256:dbl[])
                  n123 = Build Array(w258) -> (w264:dbl[])
                  n124 = Bundle By Name("Y"=w264, "t0"=timestamp(0 s since 1904-01-01), "dt"=0.0) -> (w262:waveform(dbl))  [unwired: 1 in]
                  n125 = Get Date/Time In Seconds() -> (seconds since 1Jan1904=w251:timestamp)
                  n126 = Bundle By Name("Y"=w253, "t0"=w251, "dt"=0.0) -> (w248:waveform(dbl))  [unwired: 1 in]
                  n127 = Bundle By Name("Y"=w256, "t0"=w251, "dt"=0.0) -> (w249:waveform(dbl))  [unwired: 1 in]
                  n128 = Bundle(w249, w248, w262) -> (w261:T10)  [unwired: 1 in]
                  n129 = Cluster To Array(cluster=w261) -> (array=w259:waveform(dbl)[])
                  n130 = call-poly <vilib>:"Export Waveforms to Spreadsheet File.vi"("header? (write header:T)"=FALSE ("Header? (write header:T)"), "append to file? (new file:F)"=TRUE, "waveforms"=w259, "file path (dialog if empty)"="Transient Destination") -> ()  [unwired: 6 in, 2 out]
                }
              }
              frame #3 {
                n131 = cin("clr" ("Command"), "Module # 3") -> (w274:string, →"Error 4":i32)  [unwired: 2 in]
                n132 = local write "Response 3"(w274) -> ()
              }
            }
            n133 = local read "Current position"() -> (w238:dbl)
            n134 = local read "End"() -> (w239:dbl)
            n135 = Less Or Equal?(x=w238, y=w239) -> (x <= y?=w241:bool)
            n136 = case shown="False" w241 {
              frame False {
              }
              frame True {
                n137 = Stop(stop? (T)=TRUE) -> ()
              }
            }
          }
          frame "Stop " {
            n138 = Stop(stop? (T)=TRUE) -> ()
          }
          frame "Stand by", Default {
          }
        }
      }
    }
    "Error Information" <- w2
  }
